vi "Read Limits File Path.vi"(8 "error in (no error)":errorcluster, 11 "Test Number and Bin Generator in":refnum<class "Test Number and Bin Generator.lvclass">=refnum) -> (0 "error out":errorcluster, 2 "Limits File Path":path, 3 "Test Number and Bin Generator out":refnum<class "Test Number and Bin Generator.lvclass">)   [LabVIEW 2018, in "Test Number and Bin Generator.lvlib" / "Test Number and Bin Generator.lvclass"]
uses:
  Test Number and Bin Generator.lvclass
  Test Number and Bin Generator.lvclass/Test Number and Bin Generator.ctl
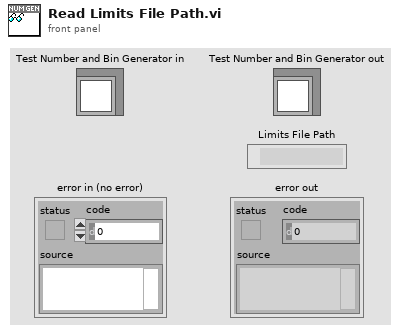
[diagram p1: front panel]
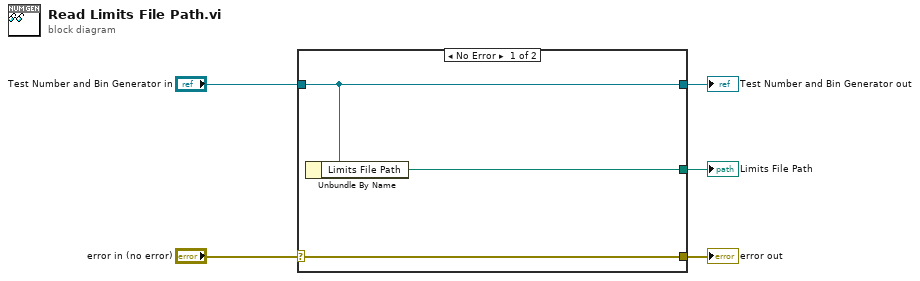
[diagram p0: block diagram]
diagram:
  n1 = case shown="No Error" "error in (no error)" {
    selector: "error in (no error)" -> [w8 w9]
    tunnel: [w8 w9] -> w4
    tunnel: [w7 w10] -> w2
    tunnel: "Test Number and Bin Generator in" -> [w7 w10]
    tunnel: [w6 _] -> w1
    frame No Error {
      n2 = Unbundle By Name(w7) -> ("Limits File Path"=w6:path)
    }
    frame Error {
    }
  }
  "error out" <- w4
  "Test Number and Bin Generator out" <- w2
  "Limits File Path" <- w1
